vi "setUiViRefnum.vi"(8 "error in (no error)":errorcluster, 10 "UI VI Refnum":refnum<vi>, 11 "Start Game in":refnum<class "Start Game.lvclass">) -> (0 "error out":errorcluster, 3 "Start Game out":refnum<class "Start Game.lvclass">)   [LabVIEW 2019, in "Start Game.lvclass"]
uses:
  Start Game.lvclass
  Start Game.lvclass/Start Game.ctl
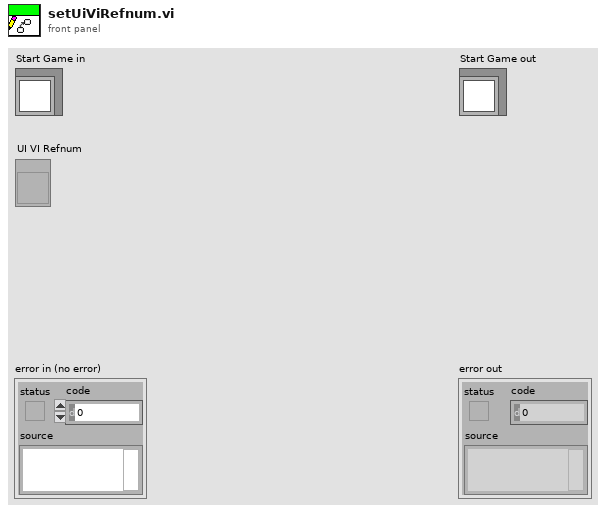
[diagram p1: front panel]
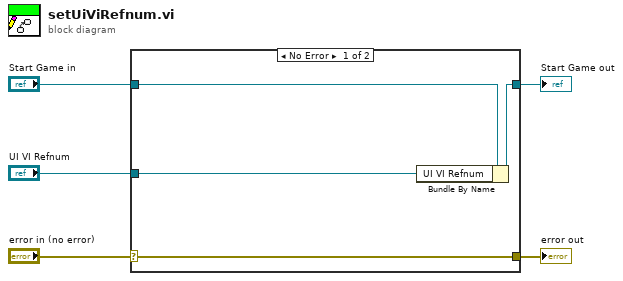
[diagram p0: block diagram]
diagram:
  n1 = case shown="No Error" "error in (no error)" {
    selector: "error in (no error)" -> [w9 w10]
    tunnel: [w9 w10] -> w4
    tunnel: [w7 w11] -> w2
    tunnel: "Start Game in" -> [w8 w11]
    tunnel: "UI VI Refnum" -> [w6 _]
    frame No Error {
      n2 = Bundle By Name(cluster=w8, "UI VI Refnum"=w6) -> (w7:refnum<class "Start Game.lvclass">)
    }
    frame Error {
    }
  }
  "error out" <- w4
  "Start Game out" <- w2
